vi "Unflatten Configuration.vi"(8 "error in (no error)":errorcluster, 10 "String":string, 11 "Configuration in":refnum<class "Configuration.lvclass">) -> (0 "error out":errorcluster, 3 "Configuration out":refnum<class "Configuration.lvclass">)   [LabVIEW 2017, in "DSF Core.lvlib" / "Configuration Session.lvclass"]
uses:
  DSF Configuration API/Configuration Session.lvclass
  Configuration.lvclass
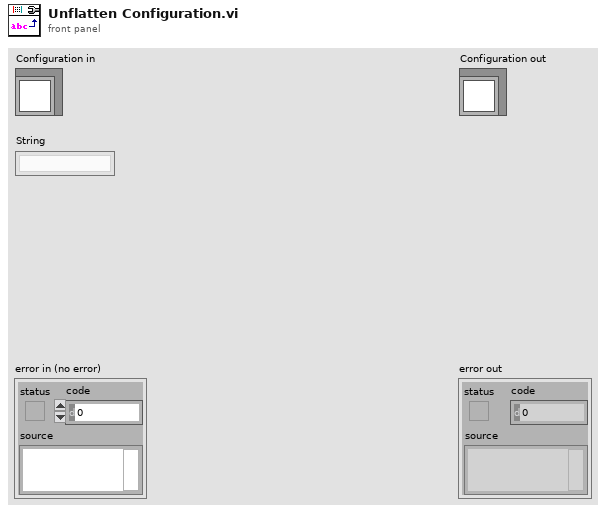
[diagram p1: front panel]
types:
  T1 = enum16{"big-endian, network order", "native, host order", "little-endian"}
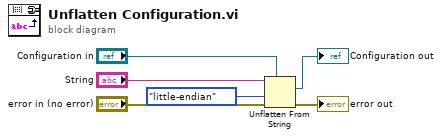
[diagram p0: block diagram]
diagram:
  n1 = Unflatten From String(type="Configuration in", binary string="String", byte order (0:big-endian, network order)=T1."little-endian", error in (no error)="error in (no error)") -> (value=→"Configuration out":refnum<class "Configuration.lvclass">, error out=→"error out":errorcluster)  [unwired: 1 in, 1 out]
